vi "PCO_SetCameraSynchMode.vi"(8 "error in (no error)":errorcluster {"code" format="%x"}, 10 "wCameraSynchMode":u16(ring) items=["OFF", "MASTER", "SLAVE"], 11 "ph":u64) -> (0 "error out":errorcluster {"code" format="%x"}, 2 "ErrorMessage":i32 format="%x", 3 "ph out":u64)   [LabVIEW 2019, in "SDK.lvlib" / "TimingControl.lvlib"]
doc: "<b>Description:</b>\nThis function does set the current camera synchronization mode. This Master / Slave synchronization mode is especially for multi-camera use.\nWhen cameras are cascaded through an external synchronization line at least one camera must be in master mode. This camera determines the timing of all other cameras in the line and therefore is the only camera, which accepts timing (exposure, delay,…) settings. All cameras which are set to slave mode synchronize its exposures with the master camera.\nSynchronization must be set to off for all cameras, which are not connected to a cascaded line.\n\nTo get reliable results the follow start / stop rules should be observed:\nIn order to get the same number of images in the recorder, please set all slaves to Recording State [run] ((see PCO_GetRecordingState), before the master is set. When setting Recording State [stop] (see PCO_GetRecordingState), please stop the master as first. Please observe the start / stop sequence.\n\n<b>Supported camera type:</b>\npco.dimax\n\n<b>Descriptor dependency:</b>\ndwGeneralCaps3: CAMERA_SYNC"
uses:
  TimingControl.lvlib
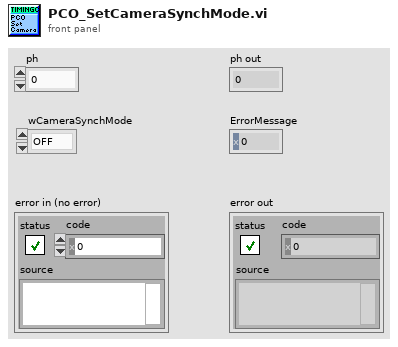
[diagram p1: front panel]
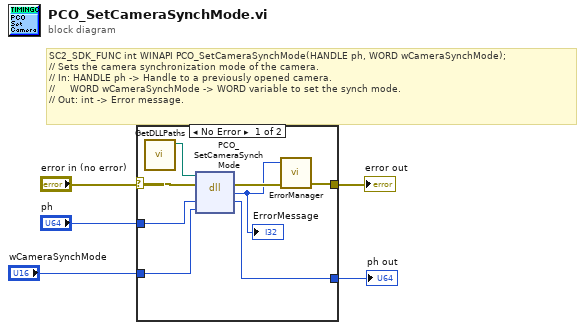
[diagram p0: block diagram]
diagram:
  # "SC2_SDK_FUNC int WINAPI PCO_SetCameraSynchMode(HANDLE ph, WORD wCameraSynchMode);\n// Sets the camera synchronization mode of the camera.\n// In: HANDLE ph -> Handle to a previously opened camera.\n//     WORD wCameraSynchMode -> WORD variable to set the synch mode.\n// Out: int -> Error message."
  n1 = case shown="No Error" "error in (no error)" {
    selector: "error in (no error)" -> [w10 w15]
    tunnel: "ph" -> [w13 w14]
    tunnel: [w12 w14] -> w4
    tunnel: "wCameraSynchMode" -> [w11 _]
    tunnel: [w8 w15] -> w2
    frame No Error {
      n2 = call "GetDLLPaths.vi"() -> ("SC2_Cam_Path"=w6:path)  [unwired: 9 in, 2 out]
      n3 = dll-call lib="?" fn="PCO_SetCameraSynchMode"(path in=w6, error in=w10, "ph"=w13, "wCameraSynchMode"=w11) -> (error out=w9:errorcluster, "return type"=w7:i32, "ph"=w12:u64)  [unwired: 2 in, 1 out]
      "ErrorMessage" <- w7
      n4 = call "ErrorManager.vi"("error in (no error)"=w9, "error code"=w7) -> ("error out"=w8:errorcluster)  [unwired: 3 in]
    }
    frame Error {
    }
  }
  "ph out" <- w4
  "error out" <- w2
